vi "DAQ_Static Dig Gen Configure and Generate.vi"(0 "DAQmx Task In":refnum<k21>, 5 "Data to Write":bool[](array[boolean]), 11 "error in":errorcluster) -> (4 "DAQmx Task Out":refnum<k21>, 6 "Channel Identifiers":refnum<k21>[](array[refnum]), 15 "error out":errorcluster)   [LabVIEW 2021, in "DAQ_Static Digital State Generation.lvlib"]
doc: "Configure, initiate, and generate static digital output data in the channels configured."
uses:
  DAQ_Static Digital State Generation.lvlib
  <vilib>/DAQmx/write.llb/DAQmx Write (Digital 1D Bool NChan 1Samp 1Line).vi
  <vilib>/DAQmx/miscellaneous.llb/DAQmx Fill In Error Info.vi
  <resource>/objmgr/daqmx.rc
panel:
  # "Inputs"
  # "Outputs"
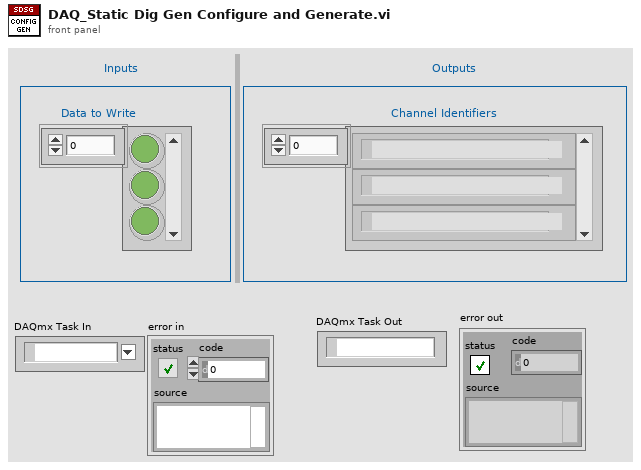
[diagram p1: front panel]
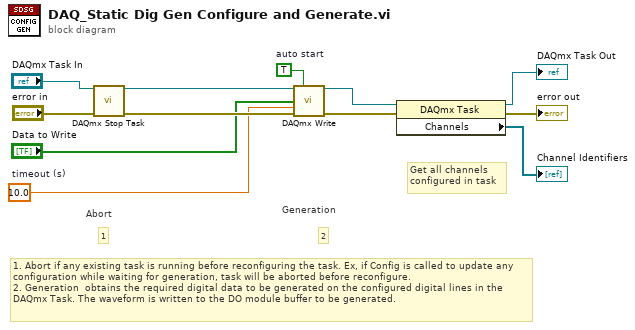
[diagram p0: block diagram]
diagram:
  w7 = TRUE  # auto start
  w6 = 10.0  # timeout (s)
  # "Get all channels\nconfigured in task"
  # "2"
  # "Generation"
  # "1"
  # "Abort"
  # "1. Abort if any existing task is running before reconfiguring the task. Ex, if Config is called to update any configuration while waiting for generation, task will be aborted before reconfigure.\n2. Generation  obtains the required digital data to be generated on the configured digital lines in the DAQmx Task. The waveform is written to the DO module buffer to be generated."
  n1 = call <vilib>:"DAQmx Stop Task.vi"("task/channels in"="DAQmx Task In", "error in"="error in") -> ("task out"=w9:refnum<k21>, "error out"=w10:errorcluster)  [unwired: 12 in]
  n2 = call-poly <vilib>:"DAQmx Write.vi"("task/channels in"=w9, "auto start"=w7, "data"="Data to Write", "timeout"=w6, "error in"=w10) -> ("task out"=w4:refnum<k21>, "error out"=w5:errorcluster)  [unwired: 8 in, 1 out]
  n3 = property class="DAQmx Task"(reference=w4, error in=w5) -> (reference out=→"DAQmx Task Out":refnum<k21>, error out=→"error out":errorcluster, "Channels"=→"Channel Identifiers":refnum<k21>[])
